vi "Instr_InitObject.vi"(8 "error in (no error)":errorcluster, 9 "Instrument Configuration":variant, 10 "Instrument address":refnum<visa-resource-name>, 11 "LXIPXISwitching in":refnum<class "LXIPXISwitching.lvclass">) -> (0 "error out":errorcluster, 3 "LXIPXISwitching out":refnum<class "LXIPXISwitching.lvclass">)   [LabVIEW 2019, in "LXIPXISwitching.lvclass"]
uses:
  LXIPXISwitching.lvclass
  InstrumentSetup.vi
  InstrControl.lvclass
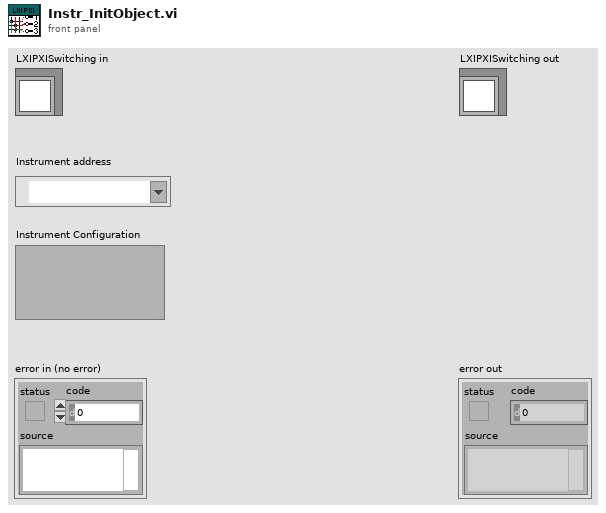
[diagram p1: front panel]
types:
  T1 = cluster{"MUX":string, "Matrix":string, "Breadboard":string, "LXIPXI Switching":refnum<class "LXIPXISwitching.lvclass">, "MUX PN":string, "Matrix  PN":string, "Breadboard PN":string, "MUX ID":string, "Matrix ID":string, "Breadboard ID":string}
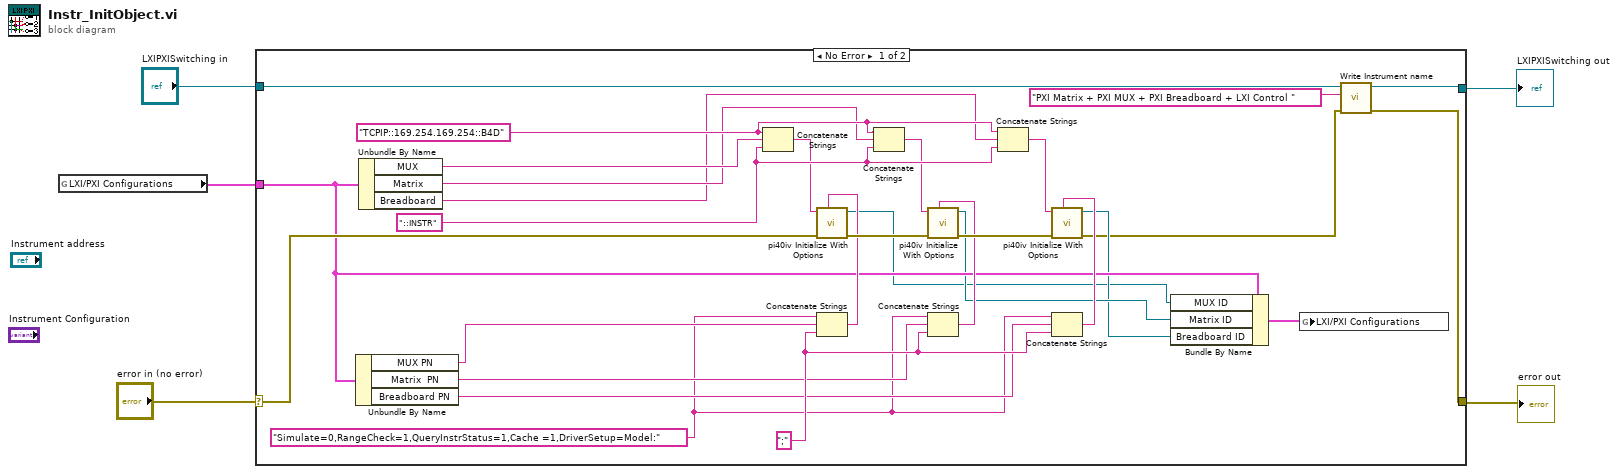
[diagram p0: block diagram]
diagram:
  n1 = global read "InstrumentSetup.vi" "LXI/PXI Configurations"() -> (w1:T1)
  n2 = case shown="No Error" "error in (no error)" {
    selector: "error in (no error)" -> [w32 w35]
    tunnel: [w7 w35] -> w4
    tunnel: [w10 w36] -> w2
    tunnel: "LXIPXISwitching in" -> [w9 w36]
    tunnel: w1 -> [w15 _]
    frame No Error {
      w23 = "TCPIP::169.254.169.254::B4D"
      w19 = "::INSTR"
      w24 = "Simulate=0,RangeCheck=1,QueryInstrStatus=1,Cache =1,DriverSetup=Model:"
      w31 = ";" ("string")
      n3 = Unbundle By Name(w15) -> ("MUX PN"=w27:string, "Matrix  PN"=w26:string, "Breadboard PN"=w25:string)
      n4 = Unbundle By Name(w15) -> ("MUX"=w22:string, "Matrix"=w21:string, "Breadboard"=w20:string)
      n5 = Concatenate Strings(w23, w22, w19) -> (w18:string)
      n6 = Concatenate Strings(w24, w27, w31) -> (w30:string)
      n7 = call <instrlib>:"pi40iv Initialize With Options.vi"("option string"=w30, "error in (no error)"=w32, "resource name"=w18) -> ("error out"=w34:errorcluster, "instrument handle out"=w11:refnum<k15>)  [unwired: 7 in]
      n8 = Concatenate Strings(w23, w21, w19) -> (w17:string)
      n9 = Concatenate Strings(w24, w26, w31) -> (w29:string)
      n10 = call <instrlib>:"pi40iv Initialize With Options.vi"("option string"=w29, "error in (no error)"=w34, "resource name"=w17) -> ("error out"=w33:errorcluster, "instrument handle out"=w14:refnum<k15>)  [unwired: 7 in]
      n11 = Concatenate Strings(w23, w20, w19) -> (w16:string)
      n12 = Concatenate Strings(w24, w25, w31) -> (w28:string)
      n13 = call <instrlib>:"pi40iv Initialize With Options.vi"("option string"=w28, "error in (no error)"=w33, "resource name"=w16) -> ("error out"=w8:errorcluster, "instrument handle out"=w13:refnum<k15>)  [unwired: 7 in]
      n14 = Bundle By Name(cluster=w15, "MUX ID"=w11, "Matrix ID"=w14, "Breadboard ID"=w13) -> (w12:T1)
      n15 = global write "InstrumentSetup.vi" "LXI/PXI Configurations"(w12) -> ()
      n16 = call-dynamic "Write Instrument name.vi"("error in (no error)"=w8, "Instrument name"="PXI Matrix + PXI MUX + PXI Breadboard + LXI Control ", "InstControl in"=w9) -> ("error out"=w7:errorcluster, "InstControl out"=w10:refnum<class "LXIPXISwitching.lvclass">)  [unwired: 7 in]
    }
    frame Error {
    }
  }
  "error out" <- w4
  "LXIPXISwitching out" <- w2
